vi "Status Created Events.vi"(11 "Base Event jettl in":refnum<class "Base Event jettl.lvclass">) -> (0 "Created Event Count":i32, 1 "Created Event Aliases":string[](array[string]), 2 "Created Event Exist?":bool, 3 "Base Event jettl out":refnum<class "Base Event jettl.lvclass">)   [LabVIEW 2021, in "jettl.lvlib" / "Base Event jettl.lvlib" / "Base Event jettl.lvclass"]
uses:
  Base Event jettl.lvclass
  Base Event jettl.lvclass/Base Event jettl.ctl
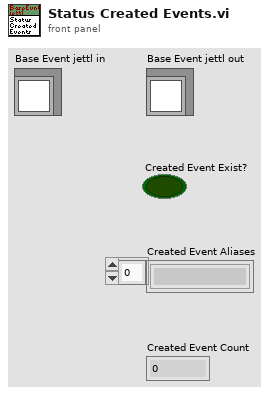
[diagram p1: front panel]
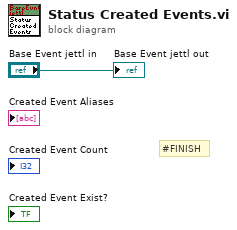
[diagram p0: block diagram]
diagram:
  # "#FINISH"
  "Base Event jettl out" <- "Base Event jettl in"
